vi "num_add.vi"   [LabVIEW 2018]
uses:
  posit.lvlib
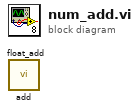
[diagram p0: block diagram]
diagram:
  n1 = call "add.vi"() -> ()  [unwired: 12 in]
  n2 = call "float_add.vi"() -> ()  [unwired: 11 in, 1 out]
